vi "GENser Wait.vi"(8 "error":errorcluster, 10 "Delay (20 mS)":u32=20, 11 "VISA":refnum<visa-resource-name>) -> (0 "error out":errorcluster, 3 "VISA out":refnum<visa-resource-name>)   [LabVIEW 2017]
doc: "Wait number of milliseconds. Used for allowing instrument to settle after changing the output. \n\nIf \"Delay\" input is not wired, there will be a 20 mSec wait.\nIf \"error\" input is set to error, the VI will not wait."
panel:
  # "Lambda Genesys \nSerial Port\n  DC Power Supplies"
  # "WAIT\nmilliSeconds"
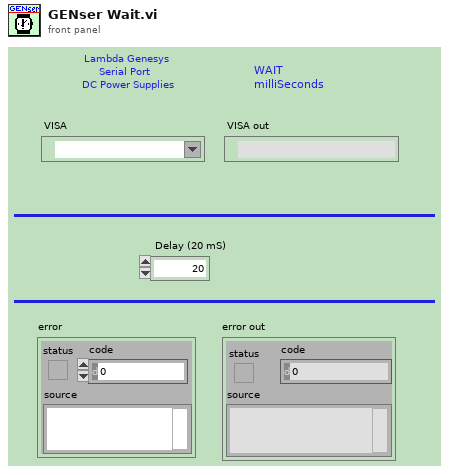
[diagram p1: front panel]
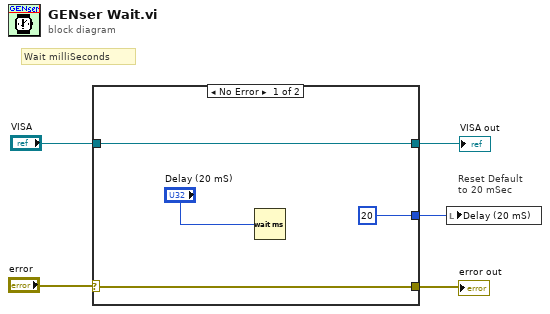
[diagram p0: block diagram]
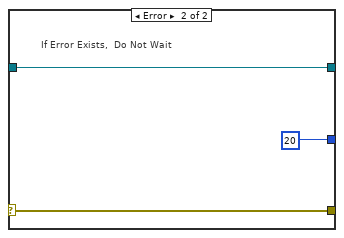
[diagram p2: hidden frame]
diagram:
  # "Reset Default\nto 20 mSec"
  # "Wait milliSeconds"
  n1 = case shown="No Error" "error" {
    selector: "error" -> [w9 w11]
    tunnel: [w9 w11] -> w4
    tunnel: "VISA" -> [w8 w12]
    tunnel: [w8 w12] -> w2
    tunnel: [u32 20 ("Delay (20 mS)") u32 20 ("Delay (20 mS)")] -> w1
    frame No Error {
      n2 = Wait (ms)(milliseconds to wait="Delay (20 mS)") -> ()  [unwired: 1 out]
    }
    frame Error {
      # "If Error Exists,  Do Not Wait"
    }
  }
  "error out" <- w4
  "VISA out" <- w2
  n3 = local write "Delay (20 mS)"(w1) -> ()
